vi "FileIOByText.vi"() -> ()   [LabVIEW 2021]
panel:
  in  "count":i32
  in  "operation (0:open)":T1(ring)
  out "Read text":string
  in  "Write text":string
  in  "Write":bool
  in  "file path (use dialog)":path
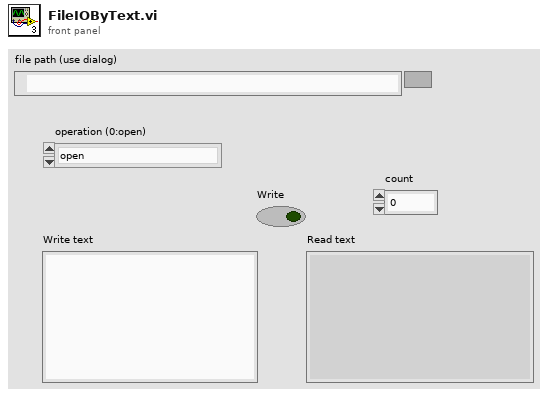
[diagram p1: front panel]
types:
  T1 = enum16{"open", "replace", "create", "open or create", "replace or create", "replace or create with confirmation"}
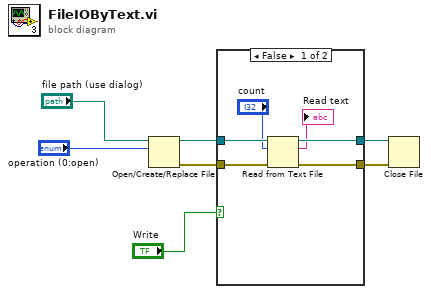
[diagram p0: block diagram]
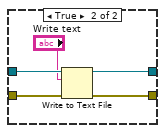
[diagram p2: hidden frame]
diagram:
  n1 = Open/Create/Replace File(file path (use dialog)="file path (use dialog)", operation (0:open)="operation (0:open)") -> (refnum out=w7:refnum<file>, error out=w6:errorcluster)  [unwired: 4 in, 1 out]
  n2 = case shown="False" "Write" {
    tunnel: w7 -> [w13 w15]
    tunnel: w6 -> [w12 w18]
    tunnel: [w11 w16] -> w5
    tunnel: [w10 w17] -> w4
    frame False {
      n3 = Read from Text File(file (use dialog)=w13, count="count", error in=w12) -> (refnum out=w11:refnum<file>, text=→"Read text":string, error out=w10:errorcluster)  [unwired: 1 in, 1 out]
    }
    frame True {
      n4 = Write to Text File(file (use dialog)=w15, text="Write text", error in=w18) -> (refnum out=w16:refnum<file>, error out=w17:errorcluster)  [unwired: 1 in, 1 out]
    }
  }
  n5 = Close File(refnum=w5, error in=w4) -> ()  [unwired: 2 out]
